vi "De-Init Lockin.vi"(8 "error in (no error)":errorcluster, 11 "DAQmx Lockin Digitizer Driver in":refnum<class "DAQmx Lockin Digitizer Driver.lvclass">) -> (0 "error out":errorcluster, 3 "DAQmx Lockin Digitizer Driver out":refnum<class "DAQmx Lockin Digitizer Driver.lvclass">)   [LabVIEW 2021, in "DAQmx Lockin Digitizer Driver.lvclass"]
uses:
  DAQmx Lockin Digitizer Driver.lvclass
  DAQmx Lockin Digitizer Driver.lvclass/DAQmx Lockin Digitizer Driver.ctl
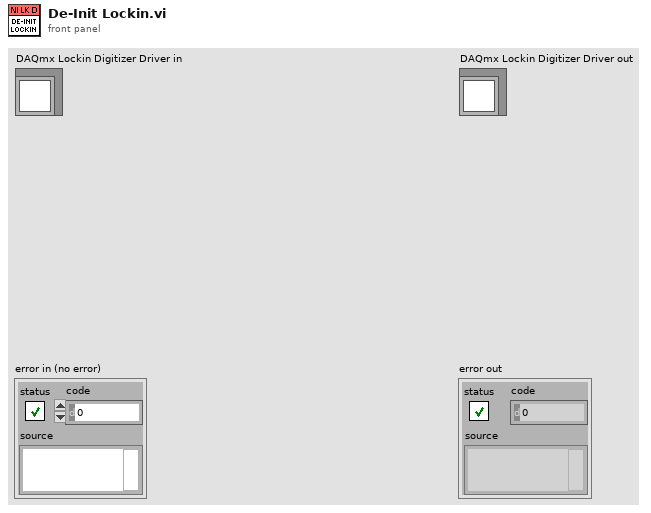
[diagram p1: front panel]
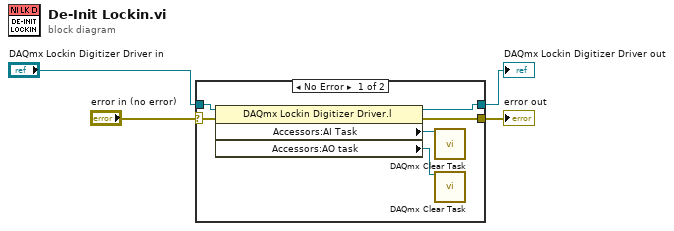
[diagram p0: block diagram]
diagram:
  n1 = case shown="No Error" "error in (no error)" {
    selector: "error in (no error)" -> [w10 w12]
    tunnel: [w9 w12] -> w3
    tunnel: [w7 w11] -> w1
    tunnel: "DAQmx Lockin Digitizer Driver in" -> [w8 w11]
    frame No Error {
      n2 = property class="DAQmx Lockin Digitizer Driver.l"(reference=w8, error in=w10) -> (reference out=w7:refnum<class "DAQmx Lockin Digitizer Driver.lvclass">, error out=w9:errorcluster, "Accessors:AI Task"=w6:refnum<k21>, "Accessors:AO task"=w5:refnum<k21>)
      n3 = call <vilib>:"DAQmx Clear Task.vi"("task in"=w6) -> ()  [unwired: 14 in, 1 out]
      n4 = call <vilib>:"DAQmx Clear Task.vi"("task in"=w5) -> ()  [unwired: 14 in, 1 out]
    }
    frame Error {
    }
  }
  "error out" <- w3
  "DAQmx Lockin Digitizer Driver out" <- w1
